vi "_Parse Measurement Error Codes.vi"(0 "String In":string) -> (1 "Reliability":i32, 2 "Results":i32[](array[numeric]))   [LabVIEW 2020, in "Rohde&Schwarz CMXP GPRF.lvlib"]
uses:
  <instrlib>/Rohde&Schwarz CMXP GPRF/Rohde&Schwarz CMXP GPRF.lvlib
  <instrlib>/Rohde&Schwarz CMXP GPRF/Private/rsidr_core.llb/rsidr_core.lvlib
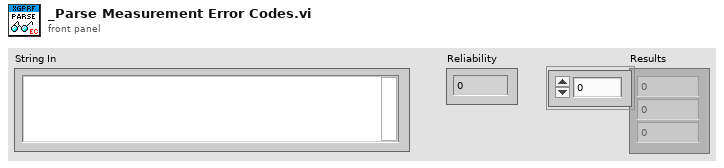
[diagram p1: front panel]
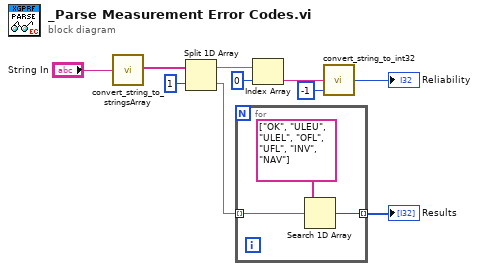
[diagram p0: block diagram]
diagram:
  n1 = call <instrlib>:"convert_string_to_stringsArray.vi"("String in"="String In") -> ("string array out"=w7:string[])  [unwired: 3 in, 1 out]
  n2 = Split 1D Array(array=w7, index=1) -> (first subarray=w5:string[], second subarray=w2:string[])
  n3 = for {
    tunnel: w2 -> [w13] mode=indexing
    tunnel: [w12] -> w1 mode=indexing
    n4 = Search 1D Array(1D array=string[] ["OK", "ULEU", "ULEL", "OFL", "UFL", "INV", "NAV"], element=w13) -> (index of element=w12:i32)  [unwired: 1 in]
  }
  "Results" <- w1
  n5 = Index Array(array=w5, index=0) -> (element=w4:string)
  n6 = call <instrlib>:"convert_string_to_int32.vi"("default (0)"=-1, "String in"=w4) -> ("int32 value out"=→"Reliability":i32)  [unwired: 3 in]
